vi "set setpoint.vi"(8 "error in (no error)":errorcluster, 10 "Setpoint":dbl[unit], 11 "VISA session":refnum<visa-resource-name>) -> (0 "error out":errorcluster, 3 "dup VISA session":refnum<visa-resource-name>)   [LabVIEW 2017]
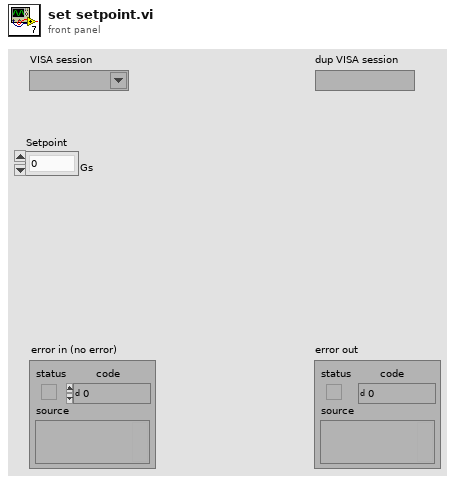
[diagram p1: front panel]
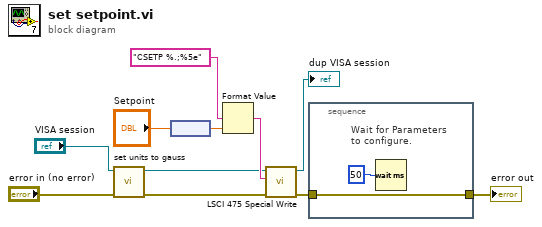
[diagram p0: block diagram]
diagram:
  n1 = call "set units to gauss.vi"("VISA session"="VISA session", "error in (no error)"="error in (no error)") -> ("dup VISA session"=w5:refnum<visa-resource-name>, "error out"=w3:errorcluster)  [unwired: 7 in]
  n2 = node("Setpoint") -> (w1:dbl)
  n3 = Format Value(format string="CSETP %.;%5e", value (0)=w1) -> (output string=w7:string)  [unwired: 1 in]
  n4 = call "LSCI 475 Special Write.vi"("error in (no error)"=w3, "Write Buffer (\"\")"=w7, "VISA session"=w5) -> ("error out"=w9:errorcluster, "dup VISA session"=→"dup VISA session":refnum<visa-resource-name>)  [unwired: 6 in, 1 out]
  n5 = stacked-sequence {
    tunnel: w9 -> [w12]
    tunnel: [w12] -> w8
    frame #0 {
      # "Wait for Parameters\nto configure."
      n6 = Wait (ms)(milliseconds to wait=u32 50) -> ()  [unwired: 1 out]
    }
  }
  "error out" <- w8
